vi "tri2.vi"(1 "Açý":string, 2 "Trigonometrik Ýþlem Türü":string) -> (0 "Sonuç":dbl)   [LabVIEW 2019]
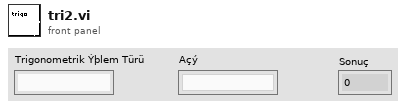
[diagram p1: front panel]
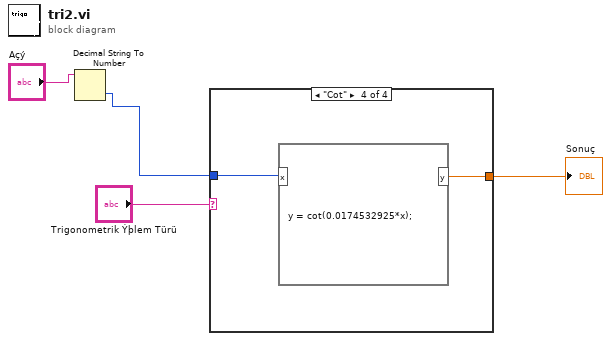
[diagram p0: block diagram]
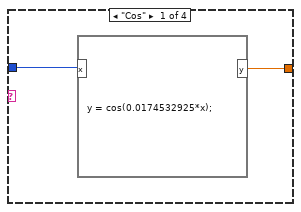
[diagram p2: hidden frame]
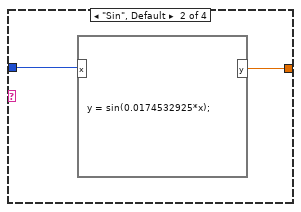
[diagram p3: hidden frame]
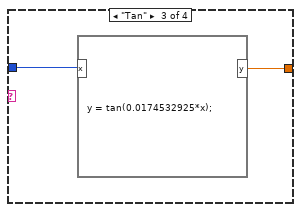
[diagram p4: hidden frame]
diagram:
  n1 = Decimal String To Number(string="Açý") -> (number=w1:i32)  [unwired: 2 in, 1 out]
  n2 = case shown="\"Cot\"" "Trigonometrik Ýþlem Türü" {
    tunnel: w1 -> [w6 w8 w10 w12]
    tunnel: [w5 w7 w9 w11] -> w3
    frame "Cos" {
      n3 = formula code="y = cos(0.0174532925*x);"("x"=w6) -> ("y"=w5:dbl)
    }
    frame "Sin", Default {
      n4 = formula code="y = sin(0.0174532925*x);"("x"=w8) -> ("y"=w7:dbl)
    }
    frame "Tan" {
      n5 = formula code="y = tan(0.0174532925*x);"("x"=w10) -> ("y"=w9:dbl)
    }
    frame "Cot" {
      n6 = formula code="y = cot(0.0174532925*x);"("x"=w12) -> ("y"=w11:dbl)
    }
  }
  "Sonuç" <- w3
